vi "write and read paths.vi"(0 "Path":string, 7 "Access":enum16{"read/write", "read-only", "write-only"}(ring), 11 "error in":errorcluster) -> (4 "Readed paths":string, 15 "error out":errorcluster)   [LabVIEW 2020, in "Custom Sort Function.lvlib"]
doc: "This VI is used to write and read paths from a text file and is used to give input to the other subVI"
uses:
  Custom Sort Function.lvlib
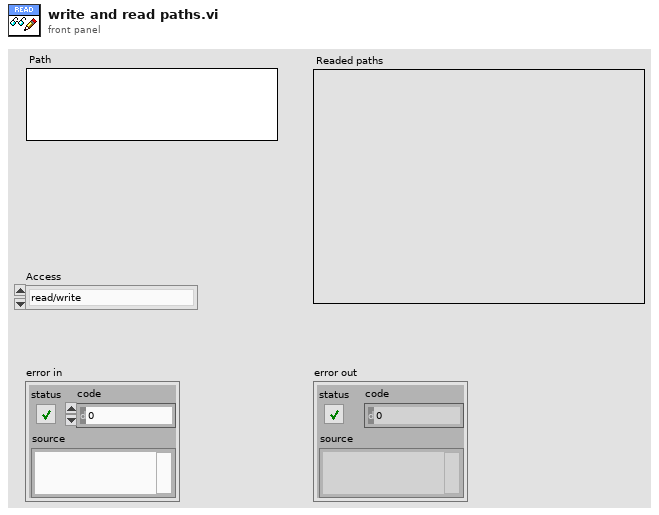
[diagram p1: front panel]
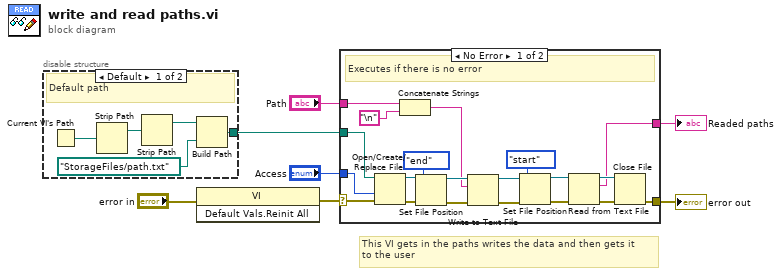
[diagram p0: block diagram]
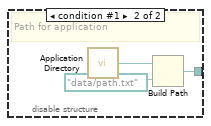
[diagram p2: hidden frame]
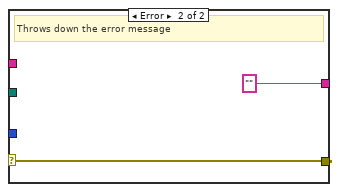
[diagram p3: hidden frame]
diagram:
  # "This VI gets in the paths writes the data and then gets it  \nto the user"
  n1 = disable-structure shown="Default" {
    disable-tunnel: [w10 w13] -> w3
    frame condition #0 (active) {
      # "Default path"
      n2 = Current VI's Path() -> (path=w12:path)
      n3 = Strip Path(path=w12) -> (stripped path=w9:path)  [unwired: 1 out]
      n4 = Strip Path(path=w9) -> (stripped path=w8:path)  [unwired: 1 out]
      n5 = Build Path(base path=w8, name or relative path=path "StorageFiles/path.txt") -> (appended path=w10:path)
    }
    frame condition #1 {
      # "Path for application"
      n6 = call <vilib>:"Application Directory.vi"() -> ("Application Directory"=w15:path)
      n7 = Build Path(base path=w15, name or relative path=path "data/path.txt") -> (appended path=w13:path)
    }
  }
  n8 = invoke class="VI" method="Default Vals.Reinit All"(error in="error in") -> (error out=w1:errorcluster)  [unwired: 2 in, 2 out]
  n9 = case shown="No Error" w1 {
    selector: w1 -> [w34 w36]
    tunnel: [w35 w36] -> w7
    tunnel: [w24 ""] -> w6
    tunnel: "Path" -> [w18 _]
    tunnel: "Access" -> [w33 _]
    tunnel: w3 -> [w32 _]
    frame No Error {
      # "Executes if there is no error"
      n10 = Open/Create/Replace File(file path (use dialog)=w32, error in=w34, access (0:read/write)=w33) -> (refnum out=w28:refnum<file>, error out=w27:errorcluster)  [unwired: 3 in, 1 out]
      n11 = Concatenate Strings(w18, "\n") -> (w16:string)
      n12 = Set File Position(refnum=w28, from (0:start)=enum16{"start", "end", "current"}."end", error in=w27) -> (refnum out=w30:refnum<file>, error out=w31:errorcluster)  [unwired: 1 in]
      n13 = Write to Text File(file (use dialog)=w30, text=w16, error in=w31) -> (refnum out=w22:refnum<file>, error out=w21:errorcluster)  [unwired: 1 in, 1 out]
      n14 = Set File Position(refnum=w22, from (0:start)=enum16{"start", "end", "current"}."start", error in=w21) -> (refnum out=w20:refnum<file>, error out=w19:errorcluster)  [unwired: 1 in]
      n15 = Read from Text File(file (use dialog)=w20, error in=w19) -> (refnum out=w25:refnum<file>, text=w24:string, error out=w26:errorcluster)  [unwired: 2 in, 1 out]
      n16 = Close File(refnum=w25, error in=w26) -> (error out=w35:errorcluster)  [unwired: 1 out]
    }
    frame Error {
      # "Throws down the error message"
    }
  }
  "error out" <- w7
  "Readed paths" <- w6
